vi "Main.vi"() -> ()   [LabVIEW 2014]
uses:
  type defs/action buttons.ctl
  type defs/mode buttons.ctl
  type defs/state.ctl
  type defs/data.ctl
  <vilib>/vision/Image Controls.llb/IMAQ Image.ctl
  type defs/task.ctl
  <vilib>/myRIO/Instrument Drivers/Onboard IO/DIO/typedefs/DIO Reference.ctl
  <vilib>/myRIO/Common/Instrument Driver Framework/Utilities/typedefs/myRIO Generic Hardware Reference.ctl
  <vilib>/myRIO/Common/Instrument Driver Framework/Utilities/typedefs/Hardware Version Enum.ctl
  <vilib>/myRIO/Common/Instrument Driver Framework/Utilities/typedefs/myRIO v1.0 Reference.ctl
  <vilib>/myRIO/Common/Instrument Driver Framework/Utilities/typedefs/Generic FPGA Reference.ctl
  <vilib>/myRIO/Common/Instrument Driver Framework/myRIO v1.0/DIO/typedefs/DIO Channels List.ctl
  <vilib>/myRIO/Common/Instrument Driver Framework/myRIO v1.0/DIO/typedefs/DIO Channels Enum.ctl
  <vilib>/userdefined/High Color/nirio_resource_hc.ctl
  <vilib>/myRIO/Common/Instrument Driver Framework/Utilities/vis/Is FPGA Ref Available.vi
  <vilib>/myRIO/Common/Instrument Driver Framework/myRIO v1.0/DIO/vis/myRIO v1.1 Open DIO.vi
  <vilib>/myRIO/Instrument Drivers/Onboard IO/DIO/vis/Write.vi
  <vilib>/myRIO/Instrument Drivers/Onboard IO/DIO/vis/Read.vi
  <vilib>/myRIO/Common/Instrument Driver Framework/Utilities/vis/Validate Channels.vi
  <vilib>/myRIO/Common/Instrument Driver Framework/myRIO v1.0/DIO/vis/myRIO v1.0 Reserve DIO.vi
  <vilib>/myRIO/Common/Instrument Driver Framework/myRIO v1.0/Resource Manager/vis/myRIO v1.0 Reserve Channel List.vi
  <vilib>/myRIO/Common/Instrument Driver Framework/myRIO v1.0/DIO/vis/myRIO v1.0 Build MUX Configuration DIO.vi
  <vilib>/myRIO/Common/Instrument Driver Framework/myRIO v1.0/Resource Manager/vis/myRIO v1.0 Reserve Channel.vi
  <vilib>/myRIO/Common/Instrument Driver Framework/myRIO v1.0/Resource Manager/vis/myRIO v1.0 Unreserve Channel.vi
  <vilib>/myRIO/Common/Instrument Driver Framework/myRIO v1.0/Resource Manager/vis/myRIO v1.0 Create Configuration List.vi
  <vilib>/myRIO/Common/Instrument Driver Framework/myRIO v1.0/Resource Manager/vis/myRIO v1.0 Build Mutex Name.vi
  <vilib>/Utility/VariantDataType/GetNumericInfo.vi
  <vilib>/Utility/error.llb/Error Cluster From Error Code.vi
  <vilib>/myRIO/Common/Instrument Driver Framework/myRIO v1.0/myRIO v1.1 Open.vi
  <vilib>/myRIO/Common/Instrument Driver Framework/Utilities/vis/IO Manager.vi
  <vilib>/myRIO/Common/Instrument Driver Framework/Utilities/vis/Configuration Manager.vi
  <vilib>/myRIO/Common/Instrument Driver Framework/myRIO v1.0/Resource Manager/vis/myRIO v1.0 Configure IO.vi
  <vilib>/myRIO/Common/Instrument Driver Framework/myRIO v1.0/myRIO v1.0 Close.vi
  <vilib>/myRIO/Common/Instrument Driver Framework/myRIO v1.0/DIO/vis/myRIO v1.0 Write DIO.vi
  <vilib>/myRIO/Common/Instrument Driver Framework/myRIO v1.0/DIO/vis/myRIO v1.0 Read DIO.vi
  <vilib>/myRIO/Express VI/Onboard Devices/LED/LED Express VI.xnode
  <vilib>/myRIO/Instrument Drivers/Onboard IO/DIO/vis/myRIO DIO Open.xnode
  <vilib>/myRIO/Express VI/Onboard Devices/Button/Button Express VI.xnode
  <vilib>/vision/NI_Vision_Development_Module.lvlib
  <vilib>/myRIO/Instrument Drivers/Onboard IO/DIO/DIO.lvlib
panel:
  in  "mode buttons":T1
  out "image display":T2(plugin-control)
  in  "action buttons":T3
  in  "Stop":bool
  # "Machine\nVision\nApp"
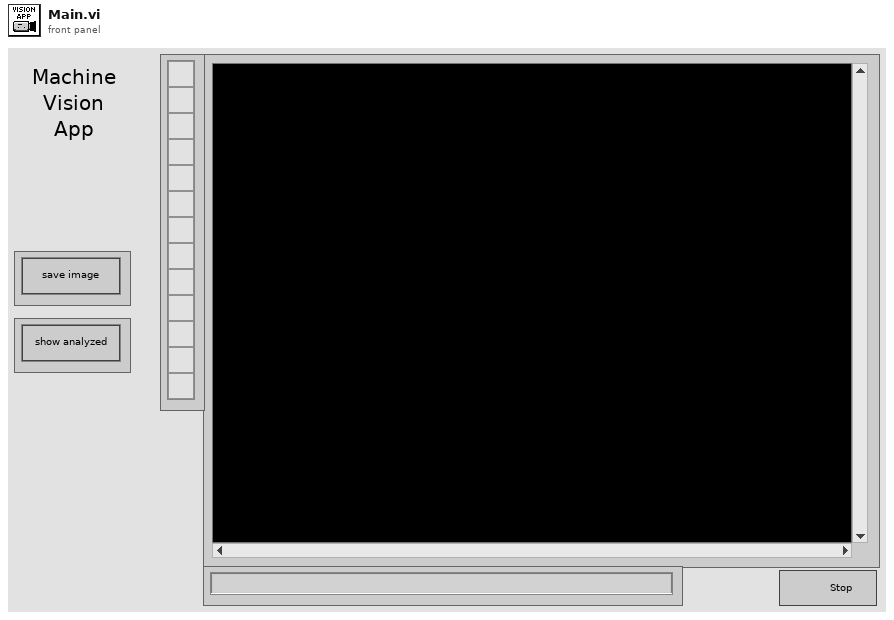
[diagram p1: front panel]
types:
  T1 = typedef "mode buttons.ctl" = cluster{"show analyzed":bool}
  T2 = typedef "IMAQ Image.ctl" = refnum<image>
  T3 = typedef "action buttons.ctl" = cluster{"save image":bool}
  T4 = typedef "data.ctl" = cluster{"save image":bool, "qsm":cluster{"Webcam image ref":T2, "Analyzed image ref":T2, "Stop webcam":bool}}
  T5 = typedef "state.ctl" = enum16{"(qsm) schedule", "(qsm) initialize", "(qsm) release", "(qsm) clean up", "(qsm) shutdown", "(myRIO) initialize", "(myRIO) clean up", "(myRIO) update ports", "(image) get", "(image) analyze", "(image) overlay", "(image) show", "save image", "state A", "state B", "state C", "state D", "state E", "state F", "state G", "state H"}
  T6 = typedef "DIO.lvlib/DIO Reference.ctl" = cluster{"myRIO Reference":T7, "DIO Channels List":T11}
  T7 = typedef "myRIO Generic Hardware Reference.ctl" = cluster{"myRIO Model":T8, "myRIO Hardware Reference":T9}
  T8 = typedef "Hardware Version Enum.ctl" = enum16{"Unknown", "myRIO-1900", "myRIO-1950"}
  T9 = typedef "myRIO v1.0 Reference.ctl" = cluster{"Generic FPGA Reference":T10, "Allow multiple opens":bool}
  T10 = typedef "Generic FPGA Reference.ctl" = refnum<k20>
  T11 = typedef "DIO Channels List.ctl" = T12[]
  T12 = typedef "DIO Channels Enum.ctl" = enum16{"Not Connected", "C/DIO0", "C/DIO1", "C/DIO2", "C/DIO3", "C/DIO4", "C/DIO5", "C/DIO6", "C/DIO7", "A/DIO0", "A/DIO1", "A/DIO2", "A/DIO3", "A/DIO4", "A/DIO5", "A/DIO6", "A/DIO7", "A/DIO8", "A/DIO9", "A/DIO10", "A/DIO11", "A/DIO12", "A/DIO13", "A/DIO14", "A/DIO15", "B/DIO0", "B/DIO1", "B/DIO2", "B/DIO3", "B/DIO4", "B/DIO5", "B/DIO6", "B/DIO7", "B/DIO8", "B/DIO9", "B/DIO10", "B/DIO11", "B/DIO12", "B/DIO13", "B/DIO14", "B/DIO15", "LED0", "LED1", "LED2", "LED3", "Button0"}
  T13 = typedef "nirio_resource_hc.ctl" = tag
  T14 = typedef "task.ctl" = T5[]
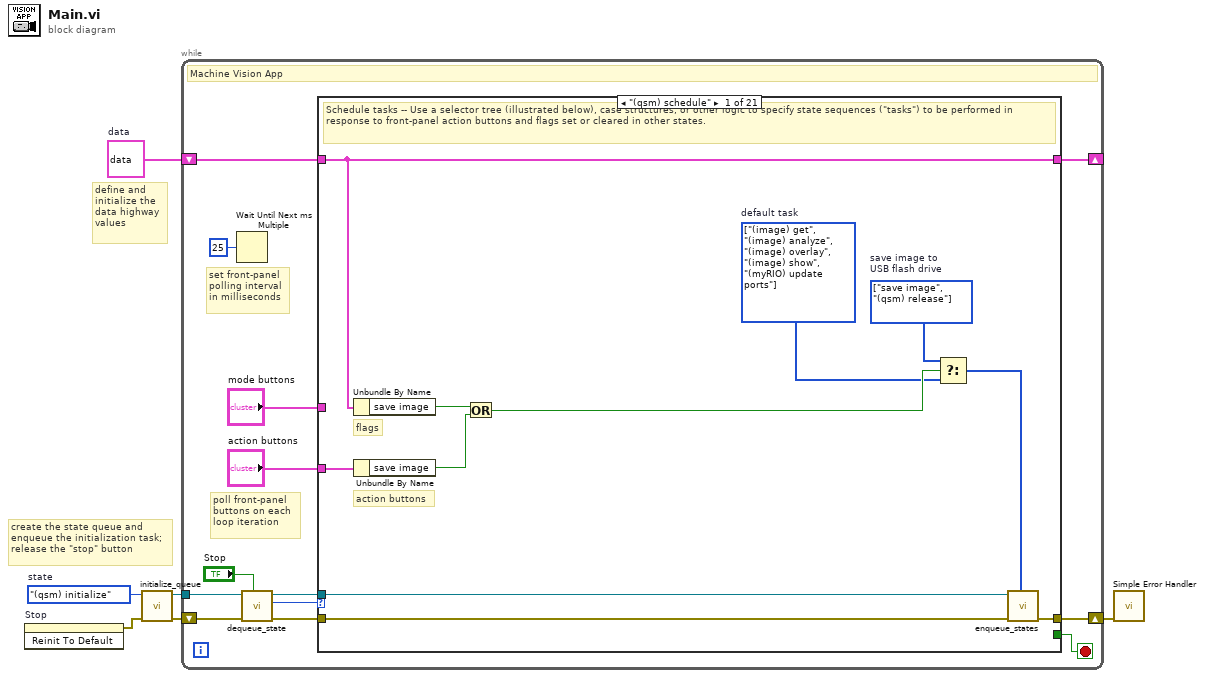
[diagram p0: block diagram]
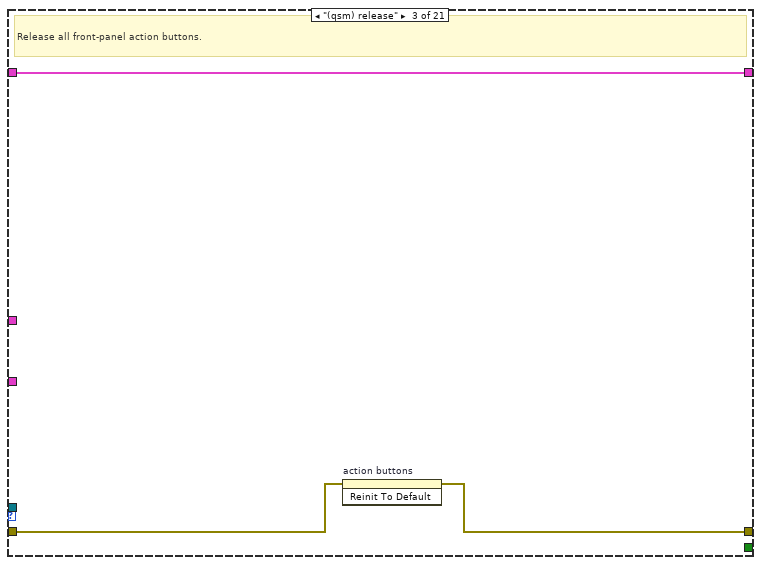
[diagram p3: hidden frame]
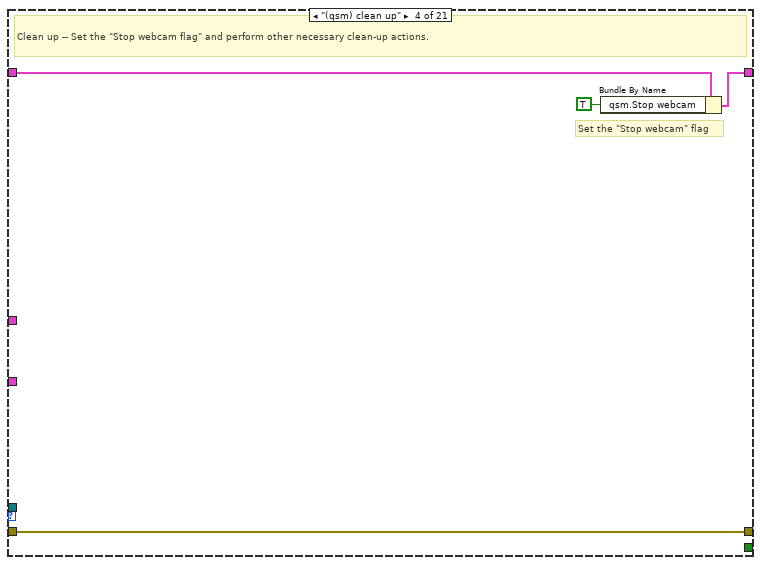
[diagram p4: hidden frame]
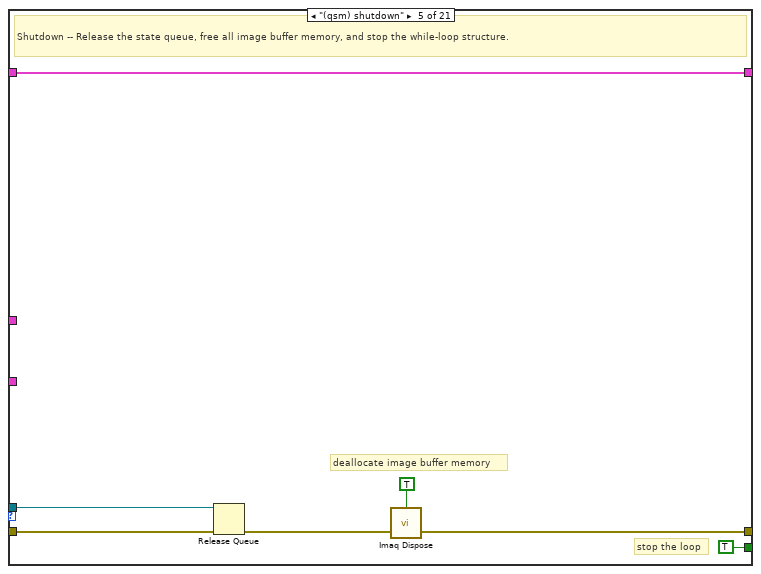
[diagram p5: hidden frame]
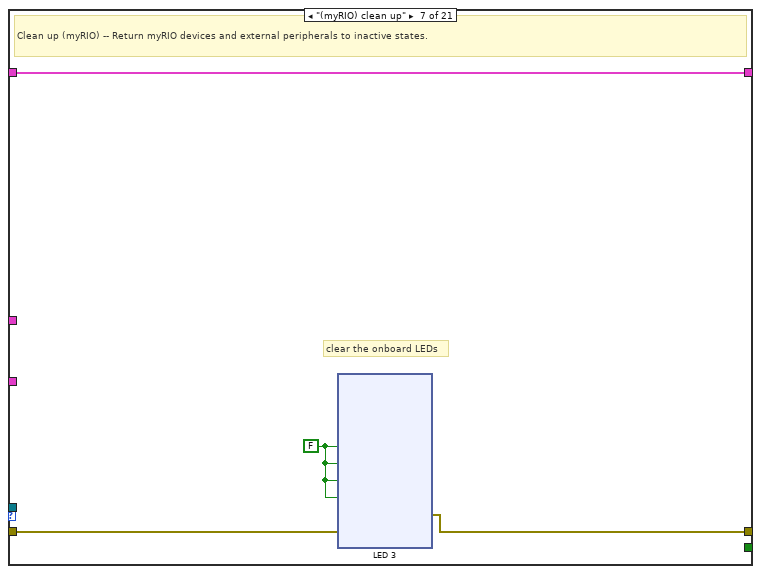
[diagram p7: hidden frame]
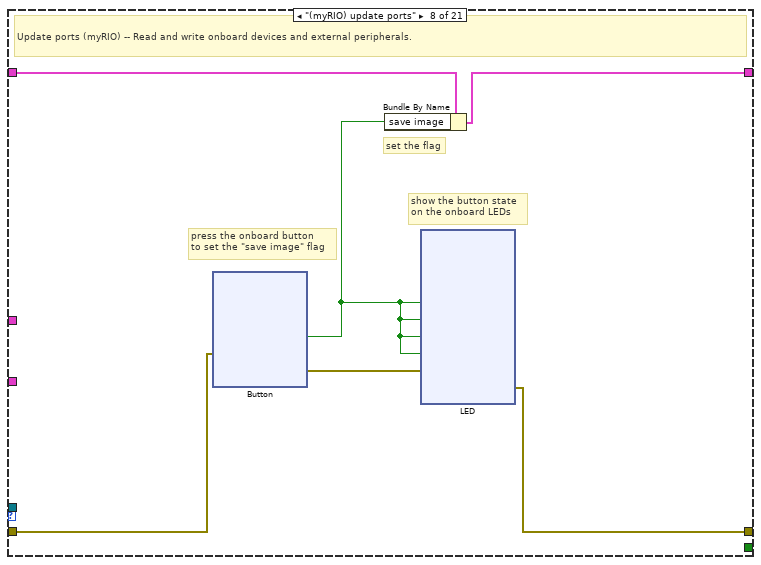
[diagram p8: hidden frame]
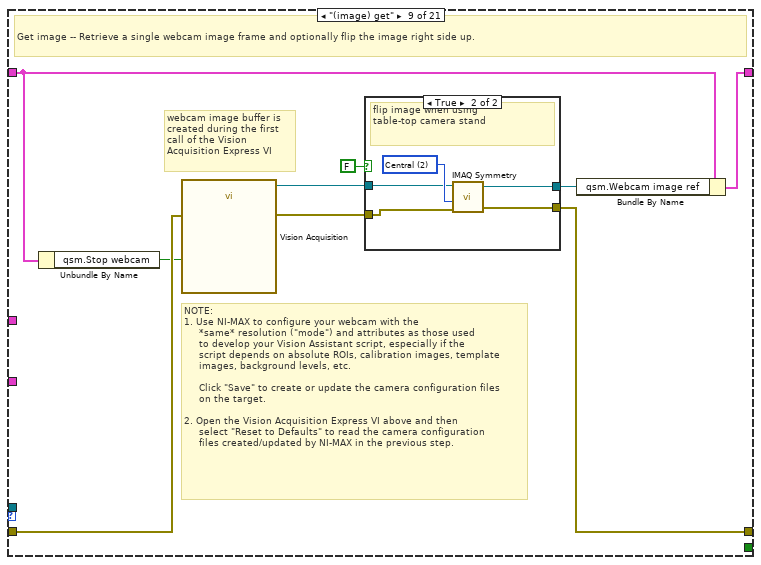
[diagram p9: hidden frame]
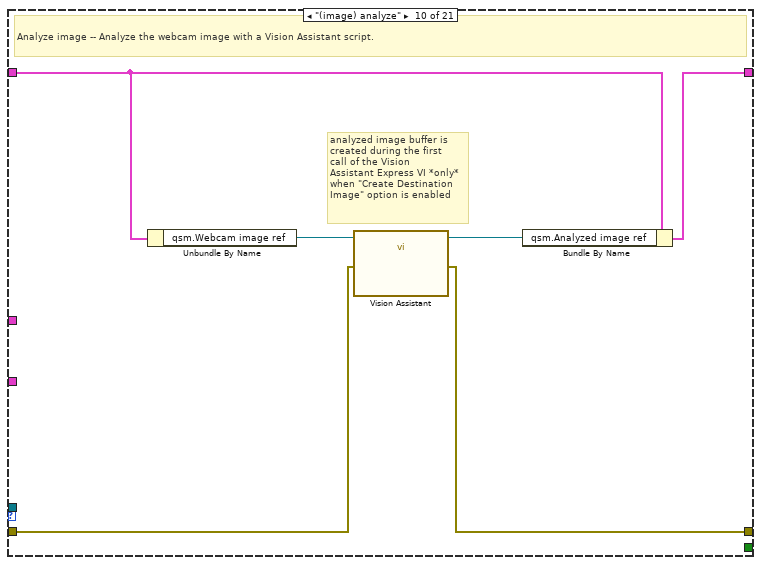
[diagram p11: hidden frame]
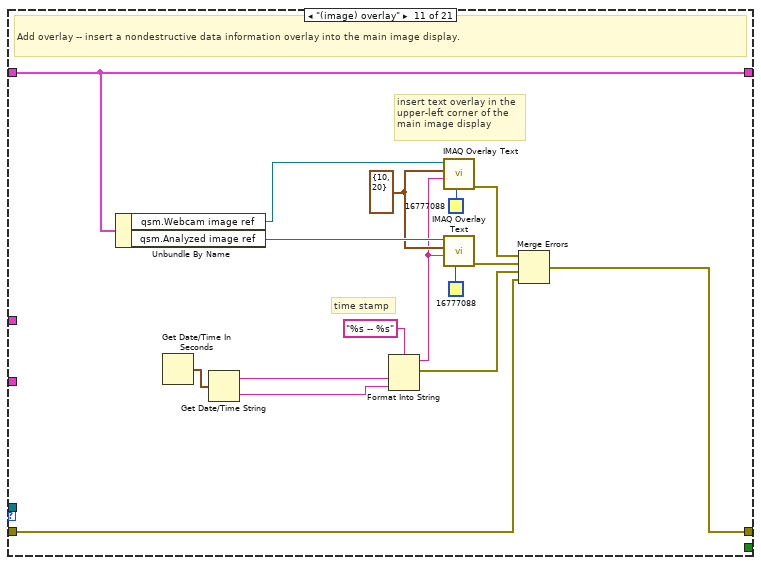
[diagram p12: hidden frame]
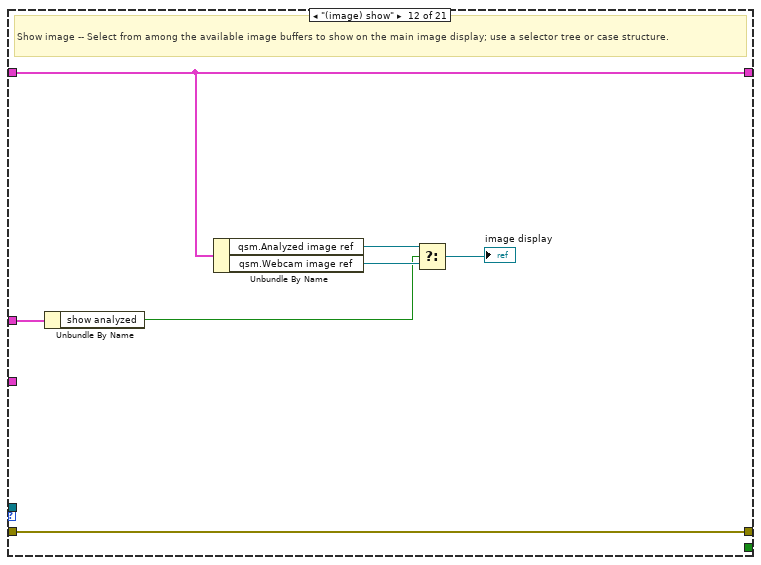
[diagram p13: hidden frame]
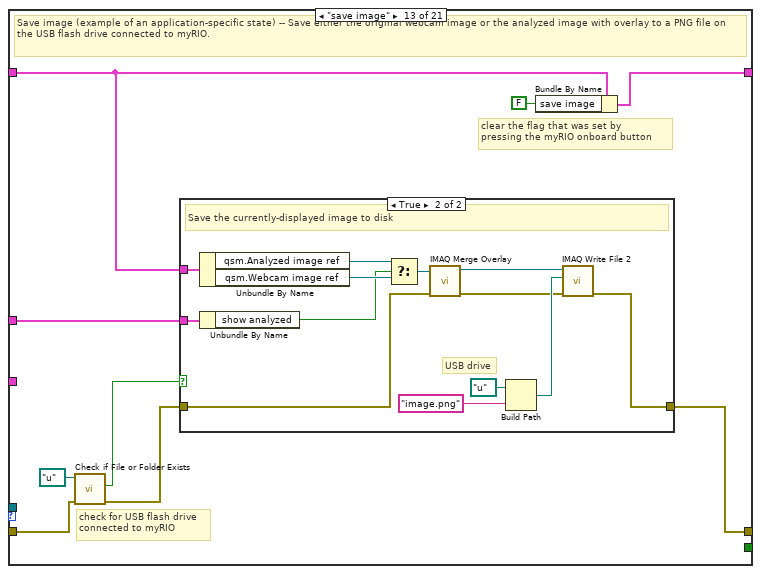
[diagram p14: hidden frame]
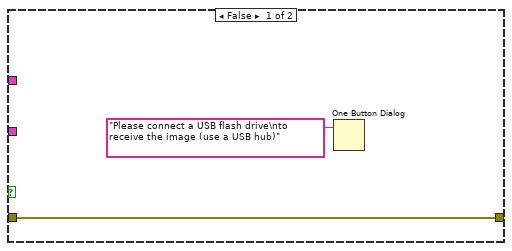
[diagram p15: hidden frame]
diagram:
  w5 = T4 {"save image"=FALSE, "qsm"={"Webcam image ref"=refnum, "Analyzed image ref"=refnum, "Stop webcam"=FALSE}}  # data
  w1 = state."(qsm) initialize"  # state
  # "define and \ninitialize the \ndata highway\nvalues"
  # "create the state queue and\nenqueue the initialization task;\nrelease the \"stop\" button"
  n1 = invoke on="Stop" class="Bool" method="Reinit To Default"() -> (error out=w2:errorcluster)  [unwired: 3 in, 2 out]
  n2 = call "initialize_queue.vi"("error in (no error)"=w2, "state"=w1) -> ("error out"=w4:errorcluster, "queue out"=w3:refnum<queue>)  [unwired: 8 in]
  n3 = while {
    shift-right: [w19] -> w6
    shift-left: w4 -> [w12]
    tunnel: w3 -> [w13]
    shift-right: [w16] -> _
    shift-left: w5 -> [w17]
    stop <- w15 stop-if-true
    # "set front-panel\npolling interval\nin milliseconds"
    # "poll front-panel\nbuttons on each\nloop iteration"
    # "Machine Vision App"
    n4 = Wait Until Next ms Multiple(millisecond multiple=u32 25) -> ()  [unwired: 1 out]
    n5 = call "dequeue_state.vi"("stop"="Stop", "error in (no error)"=w12, "queue in"=w13) -> ("error out"=w14:errorcluster, "state"=w7:T5, "queue out"=w10:refnum<queue>)  [unwired: 6 in]
    n6 = case shown="\"(qsm) schedule\"" w7 {
      tunnel: w14 -> [w26 w32 w34 w36 w45 w47 w50 w94 w178 w187 w192 w210 w219 w240 w242 w244 w246 w248 w249 w251 w254]
      tunnel: w10 -> [w27 _ _ _ w44 _ _ _ _ _ _ _ _ _ _ _ _ _ _ _ _]
      tunnel: [w28 w32 w33 w36 w40 w47 w49 w92 w173 w186 w201 w210 w217 w240 w242 w244 w246 w248 w249 w251 w254] -> w19
      tunnel: "action buttons" -> [w30 _ _ _ _ _ _ _ _ _ _ _ _ _ _ _ _ _ _ _ _]
      tunnel: w17 -> [w29 w31 w35 w38 w43 w48 w52 w96 w171 w191 w193 w211 w223 w239 w241 w243 w245 w247 w250 w252 w253]
      tunnel: [w29 w31 w35 w37 w43 w48 w52 w95 w177 w190 w193 w211 w222 w239 w241 w243 w245 w247 w250 w252 w253] -> w16
      tunnel: [_ _ _ _ TRUE _ _ _ _ _ _ _ _ _ _ _ _ _ _ _ _] -> w15
      tunnel: "mode buttons" -> [_ _ _ _ _ _ _ _ _ _ _ w209 w218 _ _ _ _ _ _ _ _]
      frame "(qsm) schedule" {
        w22 = T14 [enum."save image", enum."(qsm) release"] items=["(qsm) schedule", "(qsm) initialize", "(qsm) release", "(qsm) clean up", "(qsm) shutdown", "(myRIO) initialize", "(myRIO) clean up", "(myRIO) update ports", "(image) get", "(image) analyze", "(image) overlay", "(image) show", "save image", "state A", "state B", "state C", "state D", "state E", "state F", "state G", "state H"]  # save image to USB flash drive
        w20 = T14 [enum."(image) get", enum."(image) analyze", enum."(image) overlay", enum."(image) show", enum."(myRIO) update ports"] items=["(qsm) schedule", "(qsm) initialize", "(qsm) release", "(qsm) clean up", "(qsm) shutdown", "(myRIO) initialize", "(myRIO) clean up", "(myRIO) update ports", "(image) get", "(image) analyze", "(image) overlay", "(image) show", "save image", "state A", "state B", "state C", "state D", "state E", "state F", "state G", "state H"]  # default task
        # "action buttons"
        # "flags"
        # "Schedule tasks -- Use a selector tree (illustrated below), case structures, or other logic to specify state sequences (\"tasks\") to be performed in response to front-panel action buttons and flags set or cleared in other states."
        n7 = Unbundle By Name "Unbundle By Name"(w29) -> ("save image"=w25:bool)
        n8 = Unbundle By Name(w30) -> ("save image"=w24:bool)
        n9 = Or(x=w25, y=w24) -> (x .or. y?=w23:bool)
        n10 = Select(t=w22, s=w23, f=w20) -> (s? t:f=w21:T14)
        n11 = call "enqueue_states.vi"("task"=w21, "error in"=w26, "queue in"=w27) -> ("error out"=w28:errorcluster)  [unwired: 7 in, 1 out]
      }
      frame "(qsm) initialize" {
        # "Initialize -- Allocate memory for additional image buffers, if necessary, and perform other one-time initialization steps."
      }
      frame "(qsm) release" {
        # "Release all front-panel action buttons."
        n12 = invoke on="action buttons" class="Clust (strict)" method="Reinit To Default"(error in=w34) -> (error out=w33:errorcluster)  [unwired: 2 in, 2 out]
      }
      frame "(qsm) clean up" {
        # "Set the \"Stop webcam\" flag"
        # "Clean up -- Set the \"Stop webcam flag\" and perform other necessary clean-up actions."
        n13 = Bundle By Name(cluster=w38, "qsm.Stop webcam"=TRUE) -> (w37:T4)
      }
      frame "(qsm) shutdown" {
        # "deallocate image buffer memory"
        # "stop the loop"
        # "Shutdown -- Release the state queue, free all image buffer memory, and stop the while-loop structure."
        n14 = Release Queue(queue=w44, error in (no error)=w45) -> (error out=w41:errorcluster)  [unwired: 1 in, 2 out]
        n15 = call "Imaq Dispose"("All Images? (No)"=TRUE, "error in (no error)"=w41) -> ("error out"=w40:errorcluster)  [unwired: 4 in]
      }
      frame "(myRIO) initialize" {
        # "Initialize (myRIO) -- Open channels, configure devices, send setup strings to peripherals, etc."
      }
      frame "(myRIO) clean up" {
        w51 = FALSE ("LED3")
        # "clear the onboard LEDs"
        # "Clean up (myRIO) -- Return myRIO devices and external peripherals to inactive states."
        n16 = xnode "LED 3"("LED0"=w51, "LED1"=w51, "LED2"=w51, "LED3"=w51, "error in (no error)"=w50) -> ("error out"=w49:errorcluster)
      }
      frame "(myRIO) update ports" {
        # "show the button state\non the onboard LEDs"
        # "set the flag"
        # "press the onboard button\nto set the \"save image\" flag"
        # "Update ports (myRIO) -- Read and write onboard devices and external peripherals."
        n17 = xnode "Button"("error in (no error)"=w94) -> ("Value"=w91:bool, "error out"=w93:errorcluster)
        n18 = Bundle By Name "Bundle By Name"(cluster=w96, "save image"=w91) -> (w95:T4)
        n19 = xnode "LED"("LED0"=w91, "LED1"=w91, "LED2"=w91, "LED3"=w91, "error in (no error)"=w93) -> ("error out"=w92:errorcluster)
      }
      frame "(image) get" {
        # "webcam image buffer is\ncreated during the first\ncall of the Vision\nAcquisition Express VI"
        # "NOTE:\n1. Use NI-MAX to configure your webcam with the\n     *same* resolution (\"mode\") and attributes as those used \n     to develop your Vision Assistant script, especially if the\n     script depends on absolute ROIs, calibration images, template\n     images, background levels, etc.\n \n     Click \"Save\" to create or update the camera configuration files\n     on the target.\n\n2. Open the Vision Acquisition Express VI above and then\n     select \"Reset to Defaults\" to read the camera configuration\n     files created/updated by NI-MAX in the previous step."
        # "Get image -- Retrieve a single webcam image frame and optionally flip the image right side up."
        n20 = Unbundle By Name(w171) -> ("qsm.Stop webcam"=w170:bool)
        n21 = call "Vision Acquisition"("Stop (F)"=w170, "error in"=w178) -> ("Image Out"=w176:T2, "error out"=w174:errorcluster)  [unwired: 23 in, 1 out]
        n22 = case shown="True" FALSE {
          tunnel: w176 -> [w180 w184]
          tunnel: [w180 w183] -> w175
          tunnel: w174 -> [w179 w182]
          tunnel: [w179 w181] -> w173
          frame False {
            # "use webcam image as-is"
          }
          frame True {
            w185 = u32 2 items=["Horizontal", "Vertical", "Central", "1st Diagonal", "2nd Diagonal"] ("Type of Symmetry")
            # "flip image when using\ntable-top camera stand"
            n23 = call "IMAQ Symmetry"("error in (no error)"=w182, "Type of Symmetry"=w185, "Image Src"=w184) -> ("error out"=w181:errorcluster, "Image Dst Out"=w183:T2)  [unwired: 2 in]
          }
        }
        n24 = Bundle By Name(cluster=w171, "qsm.Webcam image ref"=w175) -> (w177:T4)
      }
      frame "(image) analyze" {
        # "analyzed image buffer is\ncreated during the first\ncall of the Vision\nAssistant Express VI *only*\nwhen \"Create Destination\nImage\" option is enabled"
        # "Analyze image -- Analyze the webcam image with a Vision Assistant script."
        n25 = Unbundle By Name "Unbundle By Name"(w191) -> ("qsm.Webcam image ref"=w189:T2)
        n26 = call "Vision Assistant"("Image In"=w189, "error in"=w187) -> ("Image Out"=w188:T2, "error out"=w186:errorcluster)  [unwired: 24 in]
        n27 = Bundle By Name "Bundle By Name"(cluster=w191, "qsm.Analyzed image ref"=w188) -> (w190:T4)
      }
      frame "(image) overlay" {
        w203 = cluster{"X":i32, "Y":i32} {"X"=10, "Y"=20} ("Origin")
        # "time stamp"
        # "insert text overlay in the\nupper-left corner of the \nmain image display"
        # "Add overlay -- insert a nondestructive data information overlay into the main image display."
        n28 = Unbundle By Name "Unbundle By Name"(w193) -> ("qsm.Webcam image ref"=w204:T2, "qsm.Analyzed image ref"=w207:T2)
        n29 = Get Date/Time In Seconds() -> (seconds since 1Jan1904=w197:timestamp)
        n30 = Get Date/Time String(seconds (now)=w197) -> (date string=w196:string, time string=w195:string)  [unwired: 2 in]
        n31 = Format Into String "Format Into String"(format string="%s -- %s", w196, w195) -> (resulting string=w198:string, error out=w194:errorcluster)  [unwired: 2 in]
        n32 = call "IMAQ Overlay Text"("Text Color (black)"=u32 16777088, "String"=w198, "Origin"=w203, "Image"=w204) -> ("error out"=w200:errorcluster)  [unwired: 6 in, 1 out]
        n33 = call "IMAQ Overlay Text"("Text Color (black)"=u32 16777088, "String"=w198, "Origin"=w203, "Image"=w207) -> ("error out"=w202:errorcluster)  [unwired: 6 in, 1 out]
        n34 = Merge Errors "Merge Errors"(w200, w202, w194, w192) -> (w201:errorcluster)
      }
      frame "(image) show" {
        # "Show image -- Select from among the available image buffers to show on the main image display; use a selector tree or case structure."
        n35 = Unbundle By Name "Unbundle By Name"(w209) -> ("show analyzed"=w208:bool)
        n36 = Unbundle By Name "Unbundle By Name"(w211) -> ("qsm.Analyzed image ref"=w214:T2, "qsm.Webcam image ref"=w213:T2)
        n37 = Select(t=w214, s=w208, f=w213) -> (s? t:f=→"image display":T2)
      }
      frame "save image" {
        # "check for USB flash drive\nconnected to myRIO"
        # "clear the flag that was set by\npressing the myRIO onboard button"
        # "Save image (example of an application-specific state) -- Save either the original webcam image or the analyzed image with overlay to a PNG file on the USB flash drive connected to myRIO."
        n38 = call <vilib>:"Check if File or Folder Exists.vi"("error in (no error)"=w219, "path"=path "u:/") -> ("error out"=w215:errorcluster, "file or folder exists?"=w216:bool)  [unwired: 7 in, 1 out]
        n39 = case shown="True" w216 {
          tunnel: w223 -> [_ w234]
          tunnel: w218 -> [_ w233]
          tunnel: [w224 w231] -> w217
          tunnel: w215 -> [w224 w229]
          frame False {
            n40 = One Button Dialog(message="Please connect a USB flash drive\nto receive the image (use a USB hub)") -> ()  [unwired: 1 in, 1 out]
          }
          frame True {
            # "USB drive"
            # "Save the currently-displayed image to disk"
            n41 = Unbundle By Name(w234) -> ("qsm.Analyzed image ref"=w228:T2, "qsm.Webcam image ref"=w235:T2)
            n42 = Unbundle By Name(w233) -> ("show analyzed"=w230:bool)
            n43 = Select(t=w228, s=w230, f=w235) -> (s? t:f=w227:T2)
            n44 = call "IMAQ Merge Overlay"("error in (no error)"=w229, "Image Src"=w227) -> ("error out"=w236:errorcluster, "Image Dst Out"=w226:T2)  [unwired: 8 in]
            n45 = Build Path(base path=path "u:/", name or relative path="image.png") -> (appended path=w237:path)
            n46 = call-poly "IMAQ Write File 2"("error in (no error)"=w236, "File Path"=w237, "Image"=w226) -> ("error out"=w231:errorcluster)  [unwired: 7 in, 1 out]
          }
        }
        n47 = Bundle By Name(cluster=w223, "save image"=FALSE) -> (w222:T4)
      }
      frame "state A" {
        # "Expansion State A"
      }
      frame "state B" {
        # "Expansion State B"
      }
      frame "state C" {
        # "Expansion State C"
      }
      frame "state D" {
        # "Expansion State D"
      }
      frame "state E" {
        # "Expansion State E"
      }
      frame "state F" {
        # "Expansion State F"
      }
      frame "state G" {
        # "Expansion State G"
      }
      frame "state H" {
        # "Expansion State H"
      }
    }
  }
  n48 = call <vilib>:"Simple Error Handler.vi"("error in (no error)"=w6) -> ()  [unwired: 4 in, 5 out]
